vi "Read MMF Header (SubVI).vi"(11 "MMF File":path) -> (0 "Header Text":string, 3 "File REF":refnum<file>)   [LabVIEW 2015]
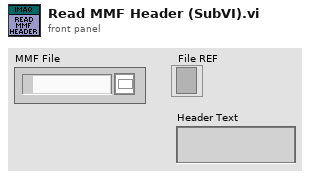
[diagram p1: front panel]
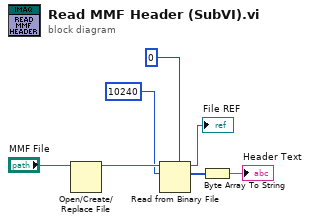
[diagram p0: block diagram]
diagram:
  n1 = Open/Create/Replace File(file path (use dialog)="MMF File") -> (refnum out=w4:refnum<file>)  [unwired: 5 in, 2 out]
  n2 = Read from Binary File(5:u8 0, 10:10240 ("count (1)"), 11:w4) -> (2:w6:u8[], 3:→"File REF":refnum<file>)  [unwired: 3 in, 2 out]
  n3 = Byte Array To String(unsigned byte array=w6) -> (string=→"Header Text":string)
